vi "On WebMessage Received.vi"(8 "error in (no error)":errorcluster, 10 "Data":T1, 11 "WebView2 Event Filter Interface in":refnum<class "WebView2 Event Filter Interface.lvclass">) -> (0 "error out":errorcluster)   [LabVIEW 2025, in "WebView2.lvlib" / "WebView2 Event Filter Interface.lvclass"]
uses:
  WebView2 Event Filter Interface.lvclass
  WebView2 Control Object/Web Message Received Event Data.ctl
  WebView2 Control Object/WebView2 Control.lvclass
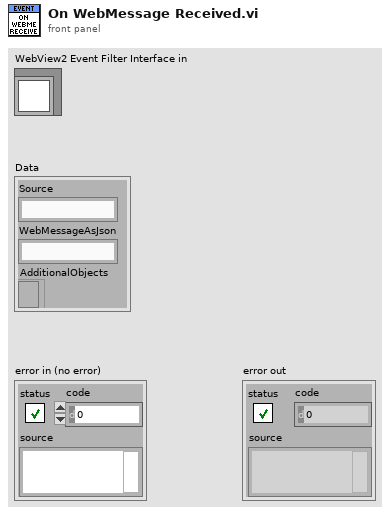
[diagram p1: front panel]
types:
  T1 = typedef "WebView2.lvlib/WebView2 Control.lvclass/Web Message Received Event Data.ctl" = cluster{"Source":string, "WebMessageAsJson":string, "AdditionalObjects":refnum<k24>}
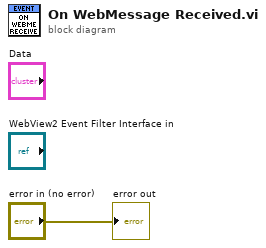
[diagram p0: block diagram]
diagram:
  "error out" <- "error in (no error)"
